vi "UpdateSingleMeasurementResult.vi"(0 "GUI_Handler_Seq in":refnum<class "GUI_Handler_Seq.lvclass">, 5 "TestMeasureStep in":refnum<class "TestMeasureStep.lvclass">, 11 "error in (no error)":errorcluster) -> (4 "GUI_Handler_Seq out":refnum<class "GUI_Handler_Seq.lvclass">, 15 "error out":errorcluster)   [LabVIEW 2017, in "GUI_Handler_Seq.lvclass"]
uses:
  GUI_Handler_Seq.lvclass
  TestMeasureStep/TestMeasureStep.lvclass
  TestMeasureStep/TestMeasureStep.lvclass/TestMeasureStep.ctl
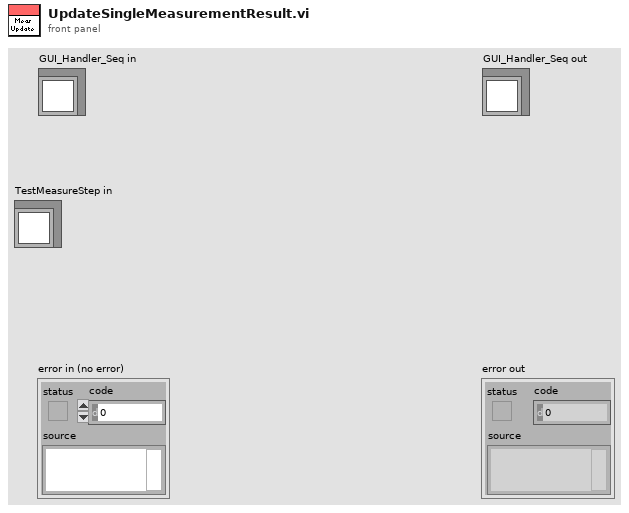
[diagram p1: front panel]
types:
  T1 = typedef "TestSeqClass.lvclass/TesstepType.ctl" = cluster{"TestName":string, "Meas":dbl, "Min ":dbl, "Max":dbl, "TestStatus":T2, "StringLimit":string, "StringMeas":string, "Unit":string}
  T2 = typedef "TestStatus.ctl" = enum16{"Not Executed", "Passed", "Failed", "Inconclusive", "Processing"}
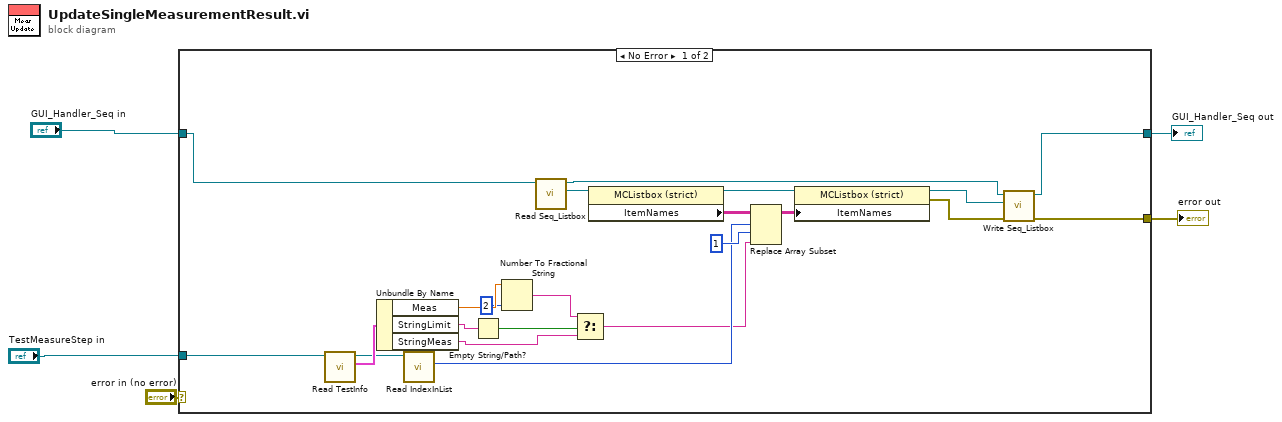
[diagram p0: block diagram]
diagram:
  n1 = case shown="No Error" "error in (no error)" {
    selector: "error in (no error)" -> [_ w29]
    tunnel: [w14 w29] -> w4
    tunnel: [w6 w28] -> w2
    tunnel: "GUI_Handler_Seq in" -> [w18 w28]
    tunnel: "TestMeasureStep in" -> [w19 _]
    frame No Error {
      n2 = call-dynamic "Read TestInfo.vi"("TestMeasureStep in"=w19) -> ("TestInfo 2"=w22:T1, "TestMeasureStep out"=w21:refnum<class "TestMeasureStep.lvclass">)  [unwired: 8 in, 1 out]
      n3 = Unbundle By Name(w22) -> ("Meas"=w11:dbl, "StringLimit"=w13:string, "StringMeas"=w8:string)
      n4 = call "Read IndexInList.vi"("TestMeasureStep in"=w21) -> ("IndexInList"=w20:u32)  [unwired: 8 in, 2 out]
      n5 = Empty String/Path?(string/path=w13) -> (empty?=w12:bool)
      n6 = Number To Fractional String(number=w11, precision (6)=i16 2) -> (F-format string=w9:string)  [unwired: 2 in]
      n7 = call-dynamic "Read Seq_Listbox.vi"("GUI_Handler_Seq in"=w18) -> ("Seq_Listbox"=w27:refnum<vi>, "GUI_Handler_Seq out"=w17:refnum<class "GUI_Handler_Seq.lvclass">)  [unwired: 8 in, 1 out]
      n8 = Select(t=w9, s=w12, f=w8) -> (s? t:f=w7:string)
      n9 = property class="MCListbox (strict)"(reference=w27) -> (reference out=w25:refnum<vi>, "ItemNames"=w26:string[][])  [unwired: 1 in, 1 out]
      n10 = Replace Array Subset(array=w26, new element=w7, index (row)=w20, index (col)=1 ("disabled index (col)")) -> (w24:string[][])
      n11 = property class="MCListbox (strict)"(reference=w25, "ItemNames"=w24) -> (reference out=w16:refnum<vi>, error out=w15:errorcluster)  [unwired: 1 in]
      n12 = call-dynamic "Write Seq_Listbox.vi"("error in (no error)"=w15, "Seq_Listbox"=w16, "GUI_Handler_Seq in"=w17) -> ("error out"=w14:errorcluster, "GUI_Handler_Seq out"=w6:refnum<class "GUI_Handler_Seq.lvclass">)  [unwired: 7 in]
    }
    frame Error {
    }
  }
  "error out" <- w4
  "GUI_Handler_Seq out" <- w2
